vi "FormCalibra9-joao.vi"() -> ()   [LabVIEW 2014]
uses:
  testMachine.ctl
  mainMachine.ctl
  <vilib>/Instr/_visa.llb/VISA Configure Serial Port (Instr).vi
  <vilib>/express/express shared/transition.llb/Dynamic To Waveform Array.vi
  <vilib>/express/express signal manip/GetorSetDDTAttributes/Set DDT Attributes/SetT0.vi
  <vilib>/express/express shared/transition.llb/Waveform Array To Dynamic.vi
  <vilib>/express/express signal manip/GetorSetDDTAttributes/Set DDT Attributes/Set DDT Properties.xnode
panel:
  in  "VISA Serial Port":refnum<visa-resource-name>
  out "editDistance":dbl caption="Distancia (m)" format="%#_4f"
  in  "Lower level":dbl
  in  "hysteresis":dbl format="%.2p"
  in  "level":dbl format="%.2p"
  out "rpm":bool
  out "editTotalWaitLimit":u8
  out "editCountWaitLimit":u8
  out "ledWaitState":bool caption="Wait State"
  out "sliderWaitUpperTime":u8(slide) max=50 scale=0.0..100.0
  out "slideWaitLowerTime":u8(slide) max=30 scale=0.0..100.0
  out "slideWaitTime":u8(slide) scale=0.0..100.0
  out "labelTestTime":string caption="Tempo total de ensaio"
  in  "buttonAcquisition":bool
  in  "editSetWaitTime":u8 caption="Tempo entre ciclos (s)" step=1 format="%0d"
  in  "stop":bool
  out "ledAcquireState":bool caption="Acquire State"
  out "editTotalLowerLimit":u8
  out "editCountLowerLimit":u8
  out "editTotalUpperLimit":u8
  out "editCountUpperLimit":u8
  out "ledEnsaio 3":bool
  out "ledBrakeState":bool caption="Brake State"
  out "ledExitState":bool caption="Exit State"
  out "ledMotorState":bool caption="Motor State"
  out "ledInit2State":bool caption="Init State"
  out "ledBlockState":bool caption="Block State"
  out "ledRunningState":bool caption="Running State"
  out "ledReadyState":bool caption="Ready State"
  out "ledInitState":bool caption="Init State"
  out "mainMachine":T1
  out "testMachine":T2=enum."finish"
  in  "editSetPathToFile":path
  in  "buttonStop":bool
  in  "buttonStart":bool
  out "graphForce":dynamicdata(graph)
  in  "editOffsetForce":dbl caption="Tara" min=0.0 max=100.0 step=0.1
  in  "editSetForce":dbl caption="Fator de conversão"
  out "editForce":dbl caption="Força (Kgf)" format="%#_4f"
  out "graphSpeed":dynamicdata(graph)
  in  "editSetSpeed":dbl caption="Fator de conversão"
  out "editSpeed":dbl caption="Velocidade (km/h)" format="%#_4f"
  out "editEngineSpeed":dbl caption="Rotação (RPM)" format="%#_4f"
  in  "buttonMotor":bool
  in  "buttonBrake":bool
  in  "editSetWaitLowerTime":u8 caption="Tempo de espera (s)"
  in  "editSetWaitUpperTime":u8=3 caption="Tempo de espera (s)"
  in  "editSetNumberOfCycles":u16 caption="Número de ciclos" max=999 step=1 format="%0d"
  in  "editSetLowerLimit":u32 caption="Limite inferior (km/h)"
  in  "editSetUpperLimit":u32 caption="Limite superior (km/h)"
  out "editTempB":dbl caption="Temperatura B (ºC)"
  out "editTempA":dbl caption="Temperatura A (ºC)"
  in  "editSetTempRef":dbl caption="Offset referência" step=0.01 format="%#_2f"
  out "editTempRef":dbl caption="Referência (ºC)"
  out "ledMotor":bool
  out "ledBrake":bool
  out "ledEnsaio":bool
  out "labelTotalCycle":string
  out "labelCurrentCycle":string
  out "labelSystemTitle":string
  in  "editCurrCycleCtr":u32
  in  "velocidade 2":u32
  out "velocidade":u32
  # "Bancada de Frenagem - Ensaio"
  # "Ensaio"
  # "Temperatura"
  # "Rotação"
  # "Célula de Carga"
  # "Configurações do ensaio"
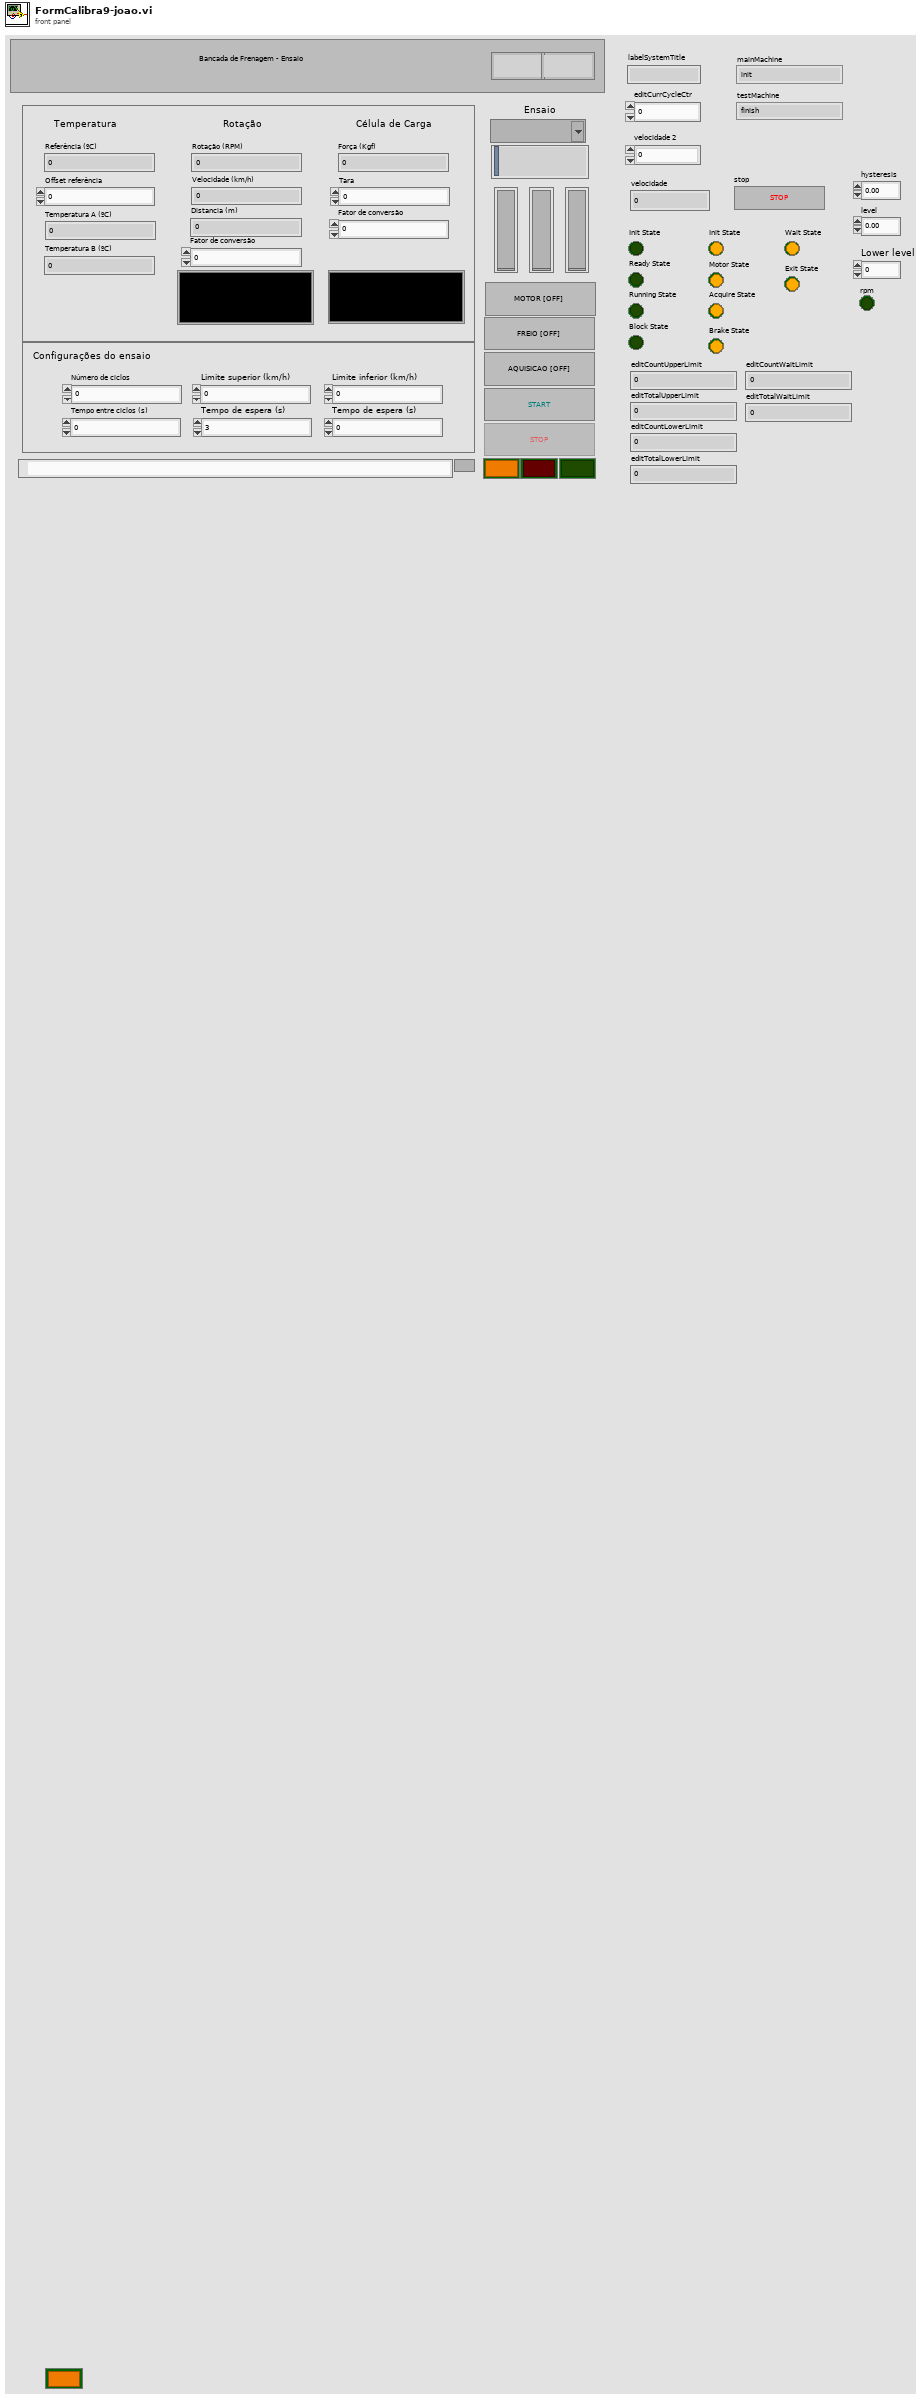
[diagram p1: front panel]
types:
  T1 = typedef "mainMachine.ctl" = enum16{"init", "ready", "running", "blocked", "finish"}
  T2 = typedef "testMachine.ctl" = enum16{"init", "motor", "motor acquire", "brake", "brake acquire", "wait ", "finish", "exit"}
  T3 = enum8{"Enabled", "Disabled", "Disabled and Grayed Out"}
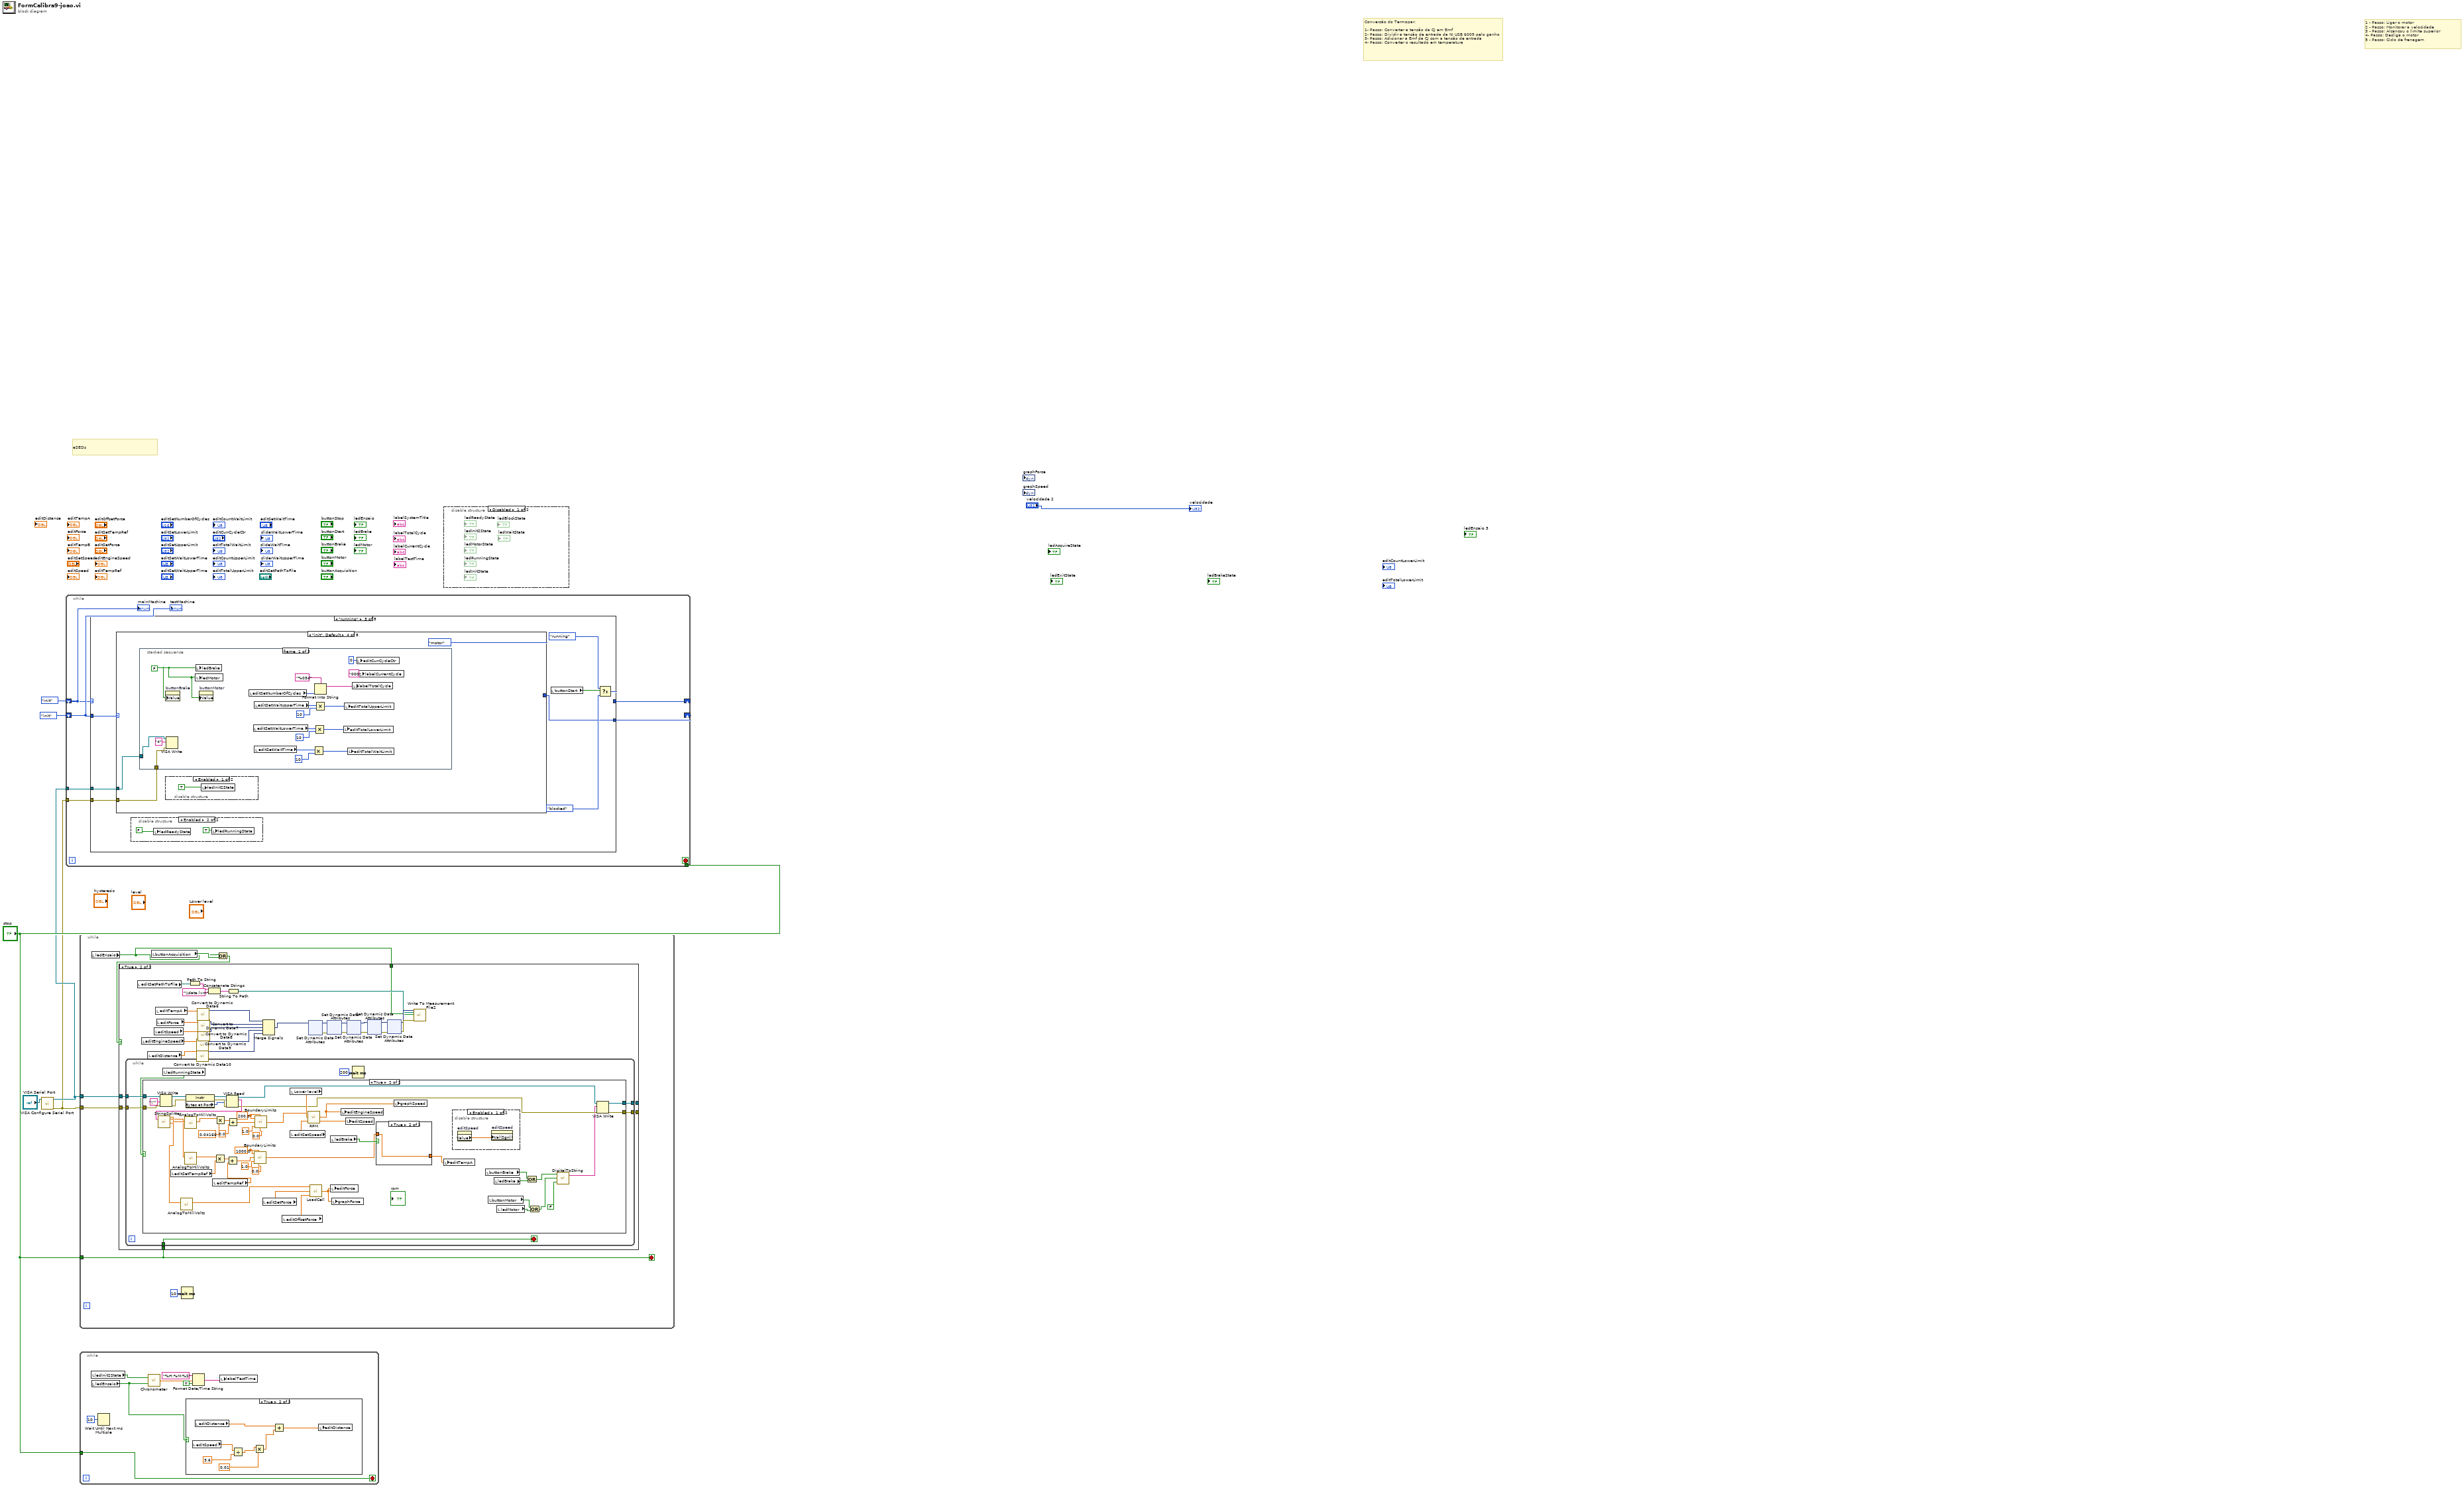
[diagram p0: block diagram]
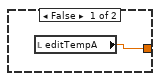
[diagram p6: hidden frame]
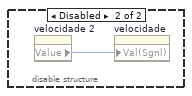
[diagram p7: hidden frame]
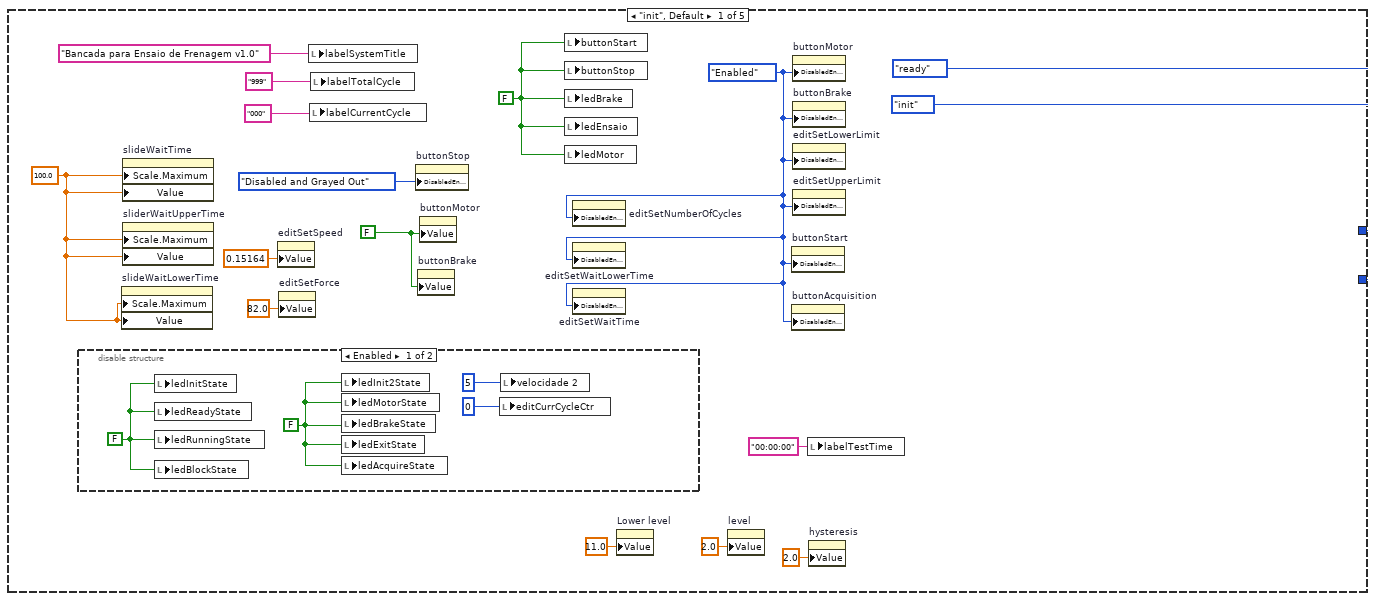
[diagram p8: hidden frame]
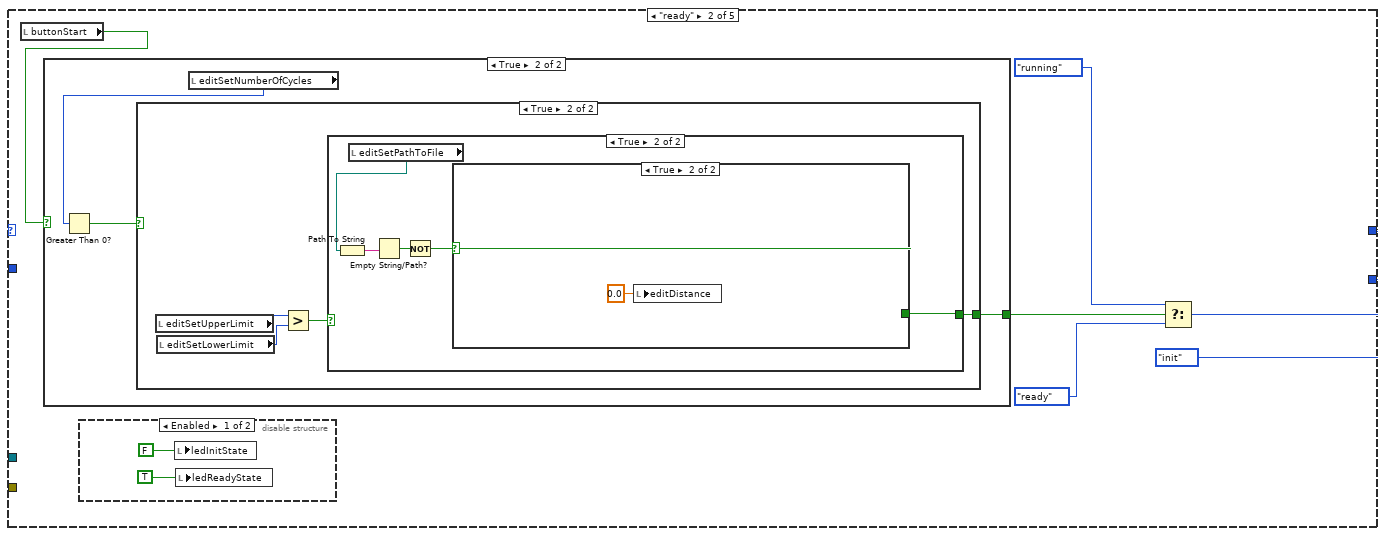
[diagram p10: hidden frame]
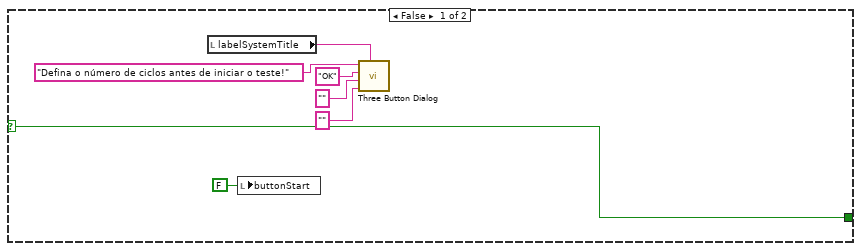
[diagram p13: hidden frame]
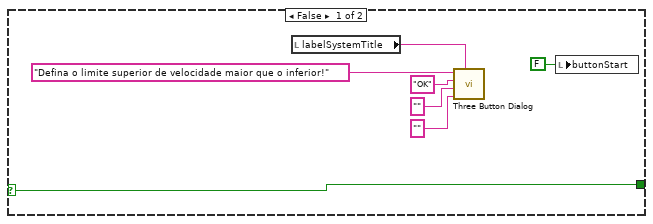
[diagram p14: hidden frame]
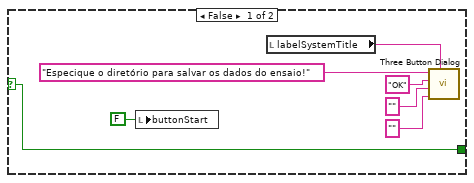
[diagram p15: hidden frame]
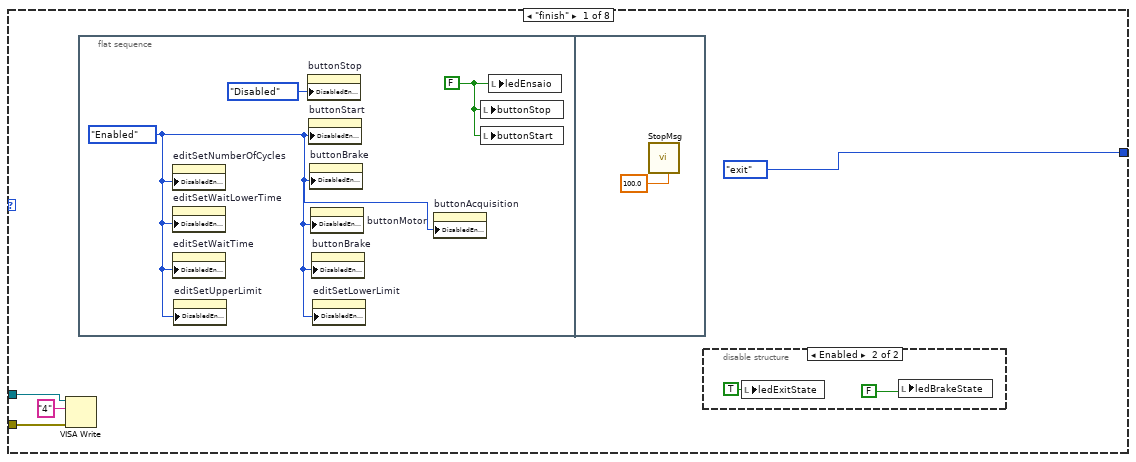
[diagram p17: hidden frame]
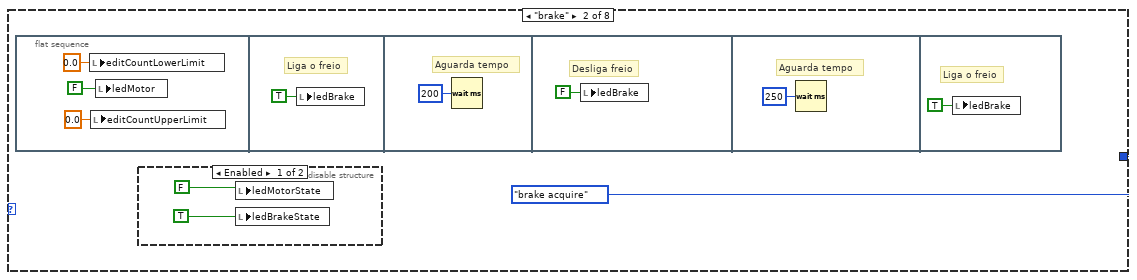
[diagram p19: hidden frame]
diagram:
  # "eSEDs"
  # "1 - Passo: Ligar o motor\n2 - Passo: Monitorar a velocidade\n3 - Passo: Alcancou o limite superior\n4- Passo: Desliga o motor\n5 - Passo: Ciclo de frenagem"
  # "Conversão do Termopar:\n\n1- Passo: Converter a tensão da CJ em Emf\n2- Passo: Dividir a tensão de entrada da NI USB 6009 pelo ganho\n3- Passo: Adicionar a Emf da CJ com a tensão de entrada\n4- Passo: Converter o resultado em temperatura"
  n1 = call-poly "VISA Configure Serial Port"("VISA resource name"="VISA Serial Port") -> ("VISA resource name out"=w3:refnum<visa-resource-name>, "error out"=w2:errorcluster)  [unwired: 13 in]
  n2 = while {
    shift-right: [w14] -> _
    shift-left: mainMachine."init" ("mainMachine") -> [w11]
    shift-right: [w13] -> _
    shift-left: testMachine."init" ("testMachine") -> [w12]
    tunnel: "stop" -> [w10]
    tunnel: w3 -> [w9]
    tunnel: w2 -> [w8]
    stop <- w10 stop-if-true
    n3 = case shown="\"running\"" w11 {
      tunnel: [mainMachine."ready" ("mainMachine") w35 w83 w235 mainMachine."finish" ("mainMachine")] -> w14
      tunnel: [testMachine."init" ("testMachine") testMachine."init" ("testMachine") w82 testMachine."init" ("testMachine") testMachine."init" ("testMachine")] -> w13
      tunnel: w12 -> [_ _ w81 _ _]
      tunnel: w9 -> [_ _ w80 _ _]
      tunnel: w8 -> [_ _ w79 _ _]
      frame "init", Default {
        w21 = 100.0 ("Scale.Range:Maximum")
        w22 = T3."Enabled" ("Disabled")
        w23 = FALSE ("buttonMotor")
        w29 = FALSE ("motor")
        n4 = disable-structure shown="Enabled" {
          frame Enabled {
            w31 = FALSE
            w32 = FALSE
            n5 = local write "ledInitState"(w32) -> ()
            n6 = local write "ledReadyState"(w32) -> ()
            n7 = local write "ledRunningState"(w32) -> ()
            n8 = local write "ledBlockState"(w32) -> ()
            n9 = local write "ledInit2State"(w31) -> ()
            n10 = local write "ledMotorState"(w31) -> ()
            n11 = local write "ledBrakeState"(w31) -> ()
            n12 = local write "ledExitState"(w31) -> ()
            n13 = local write "ledAcquireState"(w31) -> ()
            n14 = local write "editCurrCycleCtr"(u32 0 ("currentCycleCtr")) -> ()
            n15 = local write "velocidade 2"(u32 5 ("velocidade 2")) -> ()
          }
          frame Disabled {
          }
        }
        n16 = property on="slideWaitLowerTime" class="Slide (strict)"("Scale.Maximum"=w21, "Value"=w21) -> ()  [unwired: 2 in, 2 out]
        n17 = property on="slideWaitTime" class="Slide (strict)"("Scale.Maximum"=w21, "Value"=w21) -> ()  [unwired: 2 in, 2 out]
        n18 = property on="sliderWaitUpperTime" class="Slide (strict)"("Scale.Maximum"=w21, "Value"=w21) -> ()  [unwired: 2 in, 2 out]
        n19 = property on="editSetSpeed" class="DigNum (strict)"("Value"=0.15164 ("editSetSpeed")) -> ()  [unwired: 2 in, 2 out]
        n20 = property on="editSetForce" class="DigNum (strict)"("Value"=82.0 ("editSetForce")) -> ()  [unwired: 2 in, 2 out]
        n21 = local write "labelSystemTitle"("Bancada para Ensaio de Frenagem v1.0" ("systemTitle")) -> ()
        n22 = local write "labelCurrentCycle"("000" ("currentCycle")) -> ()
        n23 = local write "labelTotalCycle"("999" ("totalCycle")) -> ()
        n24 = property on="buttonStop" class="Bool (strict)"("DisabledEnum"=T3."Disabled and Grayed Out" ("Disabled")) -> ()  [unwired: 2 in, 2 out]
        n25 = property on="buttonBrake" class="Bool (strict)"("Value"=w23) -> ()  [unwired: 2 in, 2 out]
        n26 = property on="buttonMotor" class="Bool (strict)"("Value"=w23) -> ()  [unwired: 2 in, 2 out]
        n27 = local write "buttonStart"(w29) -> ()
        n28 = local write "buttonStop"(w29) -> ()
        n29 = local write "ledBrake"(w29) -> ()
        n30 = local write "ledEnsaio"(w29) -> ()
        n31 = local write "ledMotor"(w29) -> ()
        n32 = property on="editSetNumberOfCycles" class="DigNum (strict)"("DisabledEnum"=w22) -> ()  [unwired: 2 in, 2 out]
        n33 = property on="editSetWaitLowerTime" class="DigNum (strict)"("DisabledEnum"=w22) -> ()  [unwired: 2 in, 2 out]
        n34 = property on="editSetWaitTime" class="DigNum (strict)"("DisabledEnum"=w22) -> ()  [unwired: 2 in, 2 out]
        n35 = property on="Lower level" class="DigNum (strict)"("Value"=11.0 ("Lower level")) -> ()  [unwired: 2 in, 2 out]
        n36 = property on="level" class="DigNum (strict)"("Value"=2.0 ("level")) -> ()  [unwired: 2 in, 2 out]
        n37 = property on="buttonStart" class="Bool (strict)"("DisabledEnum"=w22) -> ()  [unwired: 2 in, 2 out]
        n38 = property on="buttonAcquisition" class="Bool (strict)"("DisabledEnum"=w22) -> ()  [unwired: 2 in, 2 out]
        n39 = property on="buttonMotor" class="Bool (strict)"("DisabledEnum"=w22) -> ()  [unwired: 2 in, 2 out]
        n40 = property on="buttonBrake" class="Bool (strict)"("DisabledEnum"=w22) -> ()  [unwired: 2 in, 2 out]
        n41 = property on="editSetLowerLimit" class="DigNum (strict)"("DisabledEnum"=w22) -> ()  [unwired: 2 in, 2 out]
        n42 = property on="editSetUpperLimit" class="DigNum (strict)"("DisabledEnum"=w22) -> ()  [unwired: 2 in, 2 out]
        n43 = local write "labelTestTime"("00:00:00" ("labelTestTime")) -> ()
        n44 = property on="hysteresis" class="DigNum (strict)"("Value"=2.0 ("hysteresis")) -> ()  [unwired: 2 in, 2 out]
      }
      frame "ready" {
        n45 = local read "buttonStart"() -> (w38:bool)
        n46 = case shown="True" w38 {
          selector: w38 -> [w43 _]
          tunnel: [w43 w44] -> w37
          frame False {
          }
          frame True {
            n47 = local read "editSetNumberOfCycles"() -> (w45:u16)
            n48 = Greater Than 0?(x=w45) -> (x > 0?=w46:bool)
            n49 = case shown="True" w46 {
              selector: w46 -> [w53 _]
              tunnel: [w53 w54] -> w44
              frame False {
                n50 = local read "labelSystemTitle"() -> (w48:string)
                n51 = local write "buttonStart"(FALSE ("startButton")) -> ()
                n52 = call <vilib>:"Three Button Dialog.vi"("Window Title (\"\")"=w48, "Right Button Text (\"Cancel\")"="" ("Right Button Text (\"Cancel\")"), "Center Button Text (\"No\")"="" ("Center Button Text (\"No\")"), "Left Button Text (\"Yes\")"="OK" ("Left Button Text (\"Yes\")"), "message"="Defina o número de ciclos antes de iniciar o teste!") -> ()  [unwired: 6 in, 1 out]
              }
              frame True {
                n53 = local read "editSetUpperLimit"() -> (w56:u32)
                n54 = local read "editSetLowerLimit"() -> (w55:u32)
                n55 = Greater?(x=w56, y=w55) -> (0:w57:bool)
                n56 = case shown="True" w57 {
                  selector: w57 -> [w64 _]
                  tunnel: [w64 w67] -> w54
                  frame False {
                    n57 = local read "labelSystemTitle"() -> (w59:string)
                    n58 = call <vilib>:"Three Button Dialog.vi"("Window Title (\"\")"=w59, "Right Button Text (\"Cancel\")"="" ("Right Button Text (\"Cancel\")"), "Center Button Text (\"No\")"="" ("Center Button Text (\"No\")"), "Left Button Text (\"Yes\")"="OK" ("Left Button Text (\"Yes\")"), "message"="Defina o limite superior de velocidade maior que o inferior!") -> ()  [unwired: 6 in, 1 out]
                    n59 = local write "buttonStart"(FALSE ("startButton")) -> ()
                  }
                  frame True {
                    n60 = local read "editSetPathToFile"() -> (w69:path)
                    n61 = Path To String(path=w69) -> (string=w68:string)
                    n62 = Empty String/Path?(string/path=w68) -> (empty?=w66:bool)
                    n63 = Not(x=w66) -> (.not. x?=w65:bool)
                    n64 = case shown="True" w65 {
                      selector: w65 -> [w76 w78]
                      tunnel: [w76 w78] -> w67
                      frame False {
                        n65 = local write "buttonStart"(FALSE ("startButton")) -> ()
                        n66 = local read "labelSystemTitle"() -> (w71:string)
                        n67 = call <vilib>:"Three Button Dialog.vi"("Window Title (\"\")"=w71, "Right Button Text (\"Cancel\")"="" ("Right Button Text (\"Cancel\")"), "Center Button Text (\"No\")"="" ("Center Button Text (\"No\")"), "Left Button Text (\"Yes\")"="OK" ("Left Button Text (\"Yes\")"), "message"="Especique o diretório para salvar os dados do ensaio!") -> ()  [unwired: 6 in, 1 out]
                      }
                      frame True {
                        n68 = local write "editDistance"(0.0 ("editDistance")) -> ()
                      }
                    }
                  }
                }
              }
            }
          }
        }
        n69 = disable-structure shown="Enabled" {
          frame Enabled {
            n70 = local write "ledInitState"(FALSE ("ledReady")) -> ()
            n71 = local write "ledReadyState"(TRUE ("ledReady")) -> ()
          }
          frame Disabled {
          }
        }
        n72 = Select(t=mainMachine."running" ("mainMachine"), s=w37, f=mainMachine."ready" ("mainMachine")) -> (s? t:f=w35:T1)
      }
      frame "running" {
        n73 = case shown="\"init\", Default" w81 {
          tunnel: [testMachine."exit" ("testMachine") testMachine."brake acquire" ("testMachine") testMachine."motor acquire" ("testMachine") testMachine."motor" ("testMachine") w165 w185 testMachine."exit" ("testMachine") w218] -> w82
          tunnel: w80 -> [w90 _ _ w129 _ _ _ _]
          tunnel: w79 -> [w89 _ _ w128 _ _ _ _]
          frame "finish" {
            n74 = VISA Write(VISA resource name=w90, write buffer="4", error in (no error)=w89) -> ()  [unwired: 3 out]
            n75 = flat-sequence {
              frame #0 {
                w96 = FALSE ("ledReady")
                w95 = T3."Enabled" ("Disabled")
                n76 = property on="editSetNumberOfCycles" class="DigNum (strict)"("DisabledEnum"=w95) -> ()  [unwired: 2 in, 2 out]
                n77 = property on="editSetWaitLowerTime" class="DigNum (strict)"("DisabledEnum"=w95) -> ()  [unwired: 2 in, 2 out]
                n78 = property on="editSetWaitTime" class="DigNum (strict)"("DisabledEnum"=w95) -> ()  [unwired: 2 in, 2 out]
                n79 = property on="editSetUpperLimit" class="DigNum (strict)"("DisabledEnum"=w95) -> ()  [unwired: 2 in, 2 out]
                n80 = property on="buttonStop" class="Bool (strict)"("DisabledEnum"=T3."Disabled" ("Disabled")) -> ()  [unwired: 2 in, 2 out]
                n81 = property on="buttonStart" class="Bool (strict)"("DisabledEnum"=w95) -> ()  [unwired: 2 in, 2 out]
                n82 = property on="buttonBrake" class="Bool (strict)"("DisabledEnum"=w95) -> ()  [unwired: 2 in, 2 out]
                n83 = property on="buttonMotor" class="Bool (strict)"("DisabledEnum"=w95) -> ()  [unwired: 2 in, 2 out]
                n84 = property on="buttonBrake" class="Bool (strict)"("DisabledEnum"=w95) -> ()  [unwired: 2 in, 2 out]
                n85 = property on="editSetLowerLimit" class="DigNum (strict)"("DisabledEnum"=w95) -> ()  [unwired: 2 in, 2 out]
                n86 = property on="buttonAcquisition" class="Bool (strict)"("DisabledEnum"=w95) -> ()  [unwired: 2 in, 2 out]
                n87 = local write "buttonStop"(w96) -> ()
                n88 = local write "buttonStart"(w96) -> ()
                n89 = local write "ledEnsaio"(w96) -> ()
              }
              frame #1 {
                n90 = call "StopMsg.vi"("Max Value (100)"=100.0) -> ()  [unwired: 8 in, 2 out]
              }
            }
            n91 = disable-structure shown="Enabled" {
              frame Disabled {
              }
              frame Enabled {
                n92 = local write "ledExitState"(TRUE ("ledReady")) -> ()
                n93 = local write "ledBrakeState"(FALSE ("ledReady")) -> ()
              }
            }
          }
          frame "brake" {
            n94 = flat-sequence {
              frame #0 {
                n95 = local write "editCountLowerLimit"(0.0 ("editCountUpperLimit")) -> ()
                n96 = local write "editCountUpperLimit"(0.0 ("editCountUpperLimit")) -> ()
                n97 = local write "ledMotor"(FALSE ("motor")) -> ()
              }
              frame #1 {
                # "Liga o freio"
                n98 = local write "ledBrake"(TRUE ("freio")) -> ()
              }
              frame #2 {
                # "Aguarda tempo"
                n99 = Wait (ms)(milliseconds to wait=u32 200) -> ()  [unwired: 1 out]
              }
              frame #3 {
                # "Desliga freio"
                n100 = local write "ledBrake"(FALSE ("freio")) -> ()
              }
              frame #4 {
                # "Aguarda tempo"
                n101 = Wait (ms)(milliseconds to wait=u32 250) -> ()  [unwired: 1 out]
              }
              frame #5 {
                # "Liga o freio"
                n102 = local write "ledBrake"(TRUE ("freio")) -> ()
              }
            }
            n103 = disable-structure shown="Enabled" {
              frame Enabled {
                n104 = local write "ledMotorState"(FALSE ("ledReady")) -> ()
                n105 = local write "ledBrakeState"(TRUE ("ledReady")) -> ()
              }
              frame Disabled {
              }
            }
          }
          frame "motor" {
            n106 = flat-sequence {
              frame #0 {
                n107 = local read "editCurrCycleCtr"() -> (w115:u32)
                n108 = Increment(x=w115) -> (x+1=w114:u32)
                n109 = local write "editCurrCycleCtr"(w114) -> ()
              }
              frame #1 {
                n110 = local read "editCurrCycleCtr"() -> (w122:u32)
                n111 = local read "editTotalWaitLimit"() -> (w116:u8)
                n112 = local read "editTotalUpperLimit"() -> (w118:u8)
                n113 = local read "editTotalLowerLimit"() -> (w117:u8)
                n114 = local write "editCountLowerLimit"(u8 0 ("editCountLowerLimit")) -> ()
                n115 = local write "editCountWaitLimit"(u8 0 ("editCountWaitLimit")) -> ()
                n116 = local write "editCountUpperLimit"(u8 0 ("editCountUpperLimit")) -> ()
                n117 = Format Into String(format string="%03d", w122) -> (resulting string=w123:string)  [unwired: 2 in, 1 out]
                n118 = property on="sliderWaitUpperTime" class="Slide (strict)"("Value"=w118) -> ()  [unwired: 2 in, 2 out]
                n119 = property on="slideWaitLowerTime" class="Slide (strict)"("Value"=w117) -> ()  [unwired: 2 in, 2 out]
                n120 = property on="slideWaitTime" class="Slide (strict)"("Value"=w116) -> ()  [unwired: 2 in, 2 out]
                n121 = local write "labelCurrentCycle"(w123) -> ()
              }
              frame #2 {
                # "- Liga o motor"
                n122 = local write "ledMotor"(TRUE ("motor")) -> ()
                n123 = property on="buttonStop" class="Bool (strict)"("DisabledEnum"=T3."Enabled" ("Disabled")) -> ()  [unwired: 2 in, 2 out]
                n124 = property on="buttonStart" class="Bool (strict)"("DisabledEnum"=T3."Disabled and Grayed Out" ("Disabled")) -> ()  [unwired: 2 in, 2 out]
              }
            }
            n125 = disable-structure shown="Enabled" {
              frame Enabled {
                n126 = local write "ledInit2State"(FALSE ("ledReady")) -> ()
                n127 = local write "ledBrakeState"(FALSE ("ledReady")) -> ()
                n128 = local write "ledMotorState"(TRUE ("ledReady")) -> ()
              }
              frame Disabled {
              }
            }
          }
          frame "init", Default {
            n129 = stacked-sequence {
              tunnel: w129 -> [w133 _ _]
              tunnel: w128 -> [w132 _ _]
              frame #0 {
                w140 = FALSE ("ensaio")
                n130 = property on="buttonBrake" class="Bool (strict)"("Value"=w140) -> ()  [unwired: 2 in, 2 out]
                n131 = VISA Write(VISA resource name=w133, write buffer="4", error in (no error)=w132) -> ()  [unwired: 3 out]
                n132 = local write "ledMotor"(w140) -> ()
                n133 = local write "ledBrake"(w140) -> ()
                n134 = property on="buttonMotor" class="Bool (strict)"("Value"=w140) -> ()  [unwired: 2 in, 2 out]
                n135 = local read "editSetNumberOfCycles"() -> (w147:u16)
                n136 = local read "editSetWaitLowerTime"() -> (w141:u8)
                n137 = local read "editSetWaitUpperTime"() -> (w144:u8)
                n138 = local read "editSetWaitTime"() -> (w135:u8)
                n139 = Multiply(x=w135, y=u32 10) -> (x*y=w136:u32)
                n140 = Multiply(x=w141, y=u32 10) -> (x*y=w139:u32)
                n141 = Format Into String(format string="%03d", w147) -> (resulting string=w148:string)  [unwired: 2 in, 1 out]
                n142 = Multiply(x=w144, y=u32 10) -> (x*y=w138:u32)
                n143 = local write "editTotalLowerLimit"(w139) -> ()
                n144 = local write "editTotalUpperLimit"(w138) -> ()
                n145 = local write "editTotalWaitLimit"(w136) -> ()
                n146 = local write "labelTotalCycle"(w148) -> ()
                n147 = local write "editCurrCycleCtr"(u32 0 ("currentCycleCtr")) -> ()
                n148 = local write "labelCurrentCycle"("000" ("currentCycle")) -> ()
              }
              frame #1 {
                w156 = T3."Disabled" ("Disabled")
                n149 = property on="editSetNumberOfCycles" class="DigNum (strict)"("DisabledEnum"=w156) -> ()  [unwired: 2 in, 2 out]
                n150 = property on="editSetWaitLowerTime" class="DigNum (strict)"("DisabledEnum"=w156) -> ()  [unwired: 2 in, 2 out]
                n151 = property on="editSetWaitTime" class="DigNum (strict)"("DisabledEnum"=w156) -> ()  [unwired: 2 in, 2 out]
                n152 = local read "editTotalUpperLimit"() -> (w159:u8)
                n153 = property on="sliderWaitUpperTime" class="Slide (strict)"("Scale.Maximum"=w159, "Scale.Minimum"=0.0 ("Scale.Range:Minimum"), "Scale.Increment"=1.0 ("Scale.Range:Increment"), "Value"=w159) -> ()  [unwired: 2 in, 2 out]
                n154 = property on="buttonAcquisition" class="Bool (strict)"("DisabledEnum"=w156) -> ()  [unwired: 2 in, 2 out]
                n155 = local read "editTotalLowerLimit"() -> (w153:u8)
                n156 = property on="slideWaitLowerTime" class="Slide (strict)"("Scale.Maximum"=w153, "Scale.Minimum"=0.0 ("Scale.Range:Minimum"), "Scale.Increment"=1.0 ("Scale.Range:Increment"), "Value"=w153) -> ()  [unwired: 2 in, 2 out]
                n157 = local read "editTotalWaitLimit"() -> (w150:u8)
                n158 = property on="slideWaitTime" class="Slide (strict)"("Scale.Maximum"=w150, "Scale.Minimum"=0.0 ("Scale.Range:Minimum"), "Scale.Increment"=1.0 ("Scale.Range:Increment"), "Value"=w150) -> ()  [unwired: 2 in, 2 out]
                n159 = call "StarMsg.vi"("Show"=TRUE, "Max Value (100)"=100.0) -> ()  [unwired: 7 in, 2 out]
                n160 = property on="buttonMotor" class="Bool (strict)"("DisabledEnum"=w156) -> ()  [unwired: 2 in, 2 out]
                n161 = property on="buttonBrake" class="Bool (strict)"("DisabledEnum"=w156) -> ()  [unwired: 2 in, 2 out]
                n162 = property on="editSetLowerLimit" class="DigNum (strict)"("DisabledEnum"=w156) -> ()  [unwired: 2 in, 2 out]
                n163 = property on="editSetUpperLimit" class="DigNum (strict)"("DisabledEnum"=w156) -> ()  [unwired: 2 in, 2 out]
              }
              frame #2 {
                n164 = local write "ledEnsaio"(TRUE ("ensaio")) -> ()
              }
            }
            n165 = disable-structure shown="Enabled" {
              frame Enabled {
                n166 = local write "ledInit2State"(TRUE ("ledReady")) -> ()
              }
              frame Disabled {
              }
            }
          }
          frame "motor acquire" {
            n167 = disable-structure shown="Enabled" {
              frame Enabled {
                n168 = local read "ledAcquireState"() -> (w174:bool)
                n169 = Not(x=w174) -> (.not. x?=w173:bool)
                n170 = local write "ledAcquireState"(w173) -> ()
              }
              frame Disabled {
              }
            }
            n171 = Wait (ms)(milliseconds to wait=u32 100) -> ()  [unwired: 1 out]
            n172 = disable-structure shown="Enabled" {
              disable-tunnel: [w171 w172] -> w164
              frame Enabled {
                n173 = property on="editSpeed" class="DigNum (strict)"() -> ("Value"=w171:dbl)  [unwired: 2 in, 2 out]
              }
              frame Disabled {
                n174 = property on="velocidade" class="DigNum (strict)"() -> ("Value"=w172:u32)  [unwired: 2 in, 2 out]
              }
            }
            n175 = property on="editSetUpperLimit" class="DigNum (strict)"() -> ("Value"=w163:u32)  [unwired: 2 in, 2 out]
            n176 = Greater Or Equal?(x=w164, y=w163) -> (x >= y?=w169:bool)
            n177 = case shown="True" w169 {
              selector: w169 -> [w175 _]
              tunnel: [w175 w176] -> w168
              frame False {
              }
              frame True {
                n178 = flat-sequence {
                  tunnel: [w181] -> w176
                  frame #0 {
                    n179 = local read "editCountUpperLimit"() -> (w179:u8)
                    n180 = Increment(x=w179) -> (x+1=w177:u8)
                    n181 = local write "editCountUpperLimit"(w177) -> ()
                    n182 = local read "editTotalUpperLimit"() -> (w178:u8)
                    n183 = Subtract(x=w178, y=w177) -> (x-y=w180:u8)
                    n184 = property on="sliderWaitUpperTime" class="Slide (strict)"("Value"=w180) -> ()  [unwired: 2 in, 2 out]
                  }
                  frame #1 {
                    n185 = local read "editCountUpperLimit"() -> (w183:u8)
                    n186 = local read "editTotalUpperLimit"() -> (w182:u8)
                    n187 = Greater Or Equal?(x=w183, y=w182) -> (x >= y?=w181:bool)
                  }
                }
              }
            }
            n188 = Select(t=testMachine."brake" ("testMachine"), s=w168, f=testMachine."motor acquire" ("testMachine")) -> (s? t:f=w165:T2)
          }
          frame "brake acquire" {
            n189 = disable-structure shown="Enabled" {
              frame Enabled {
                n190 = local read "ledAcquireState"() -> (w193:bool)
                n191 = Not(x=w193) -> (.not. x?=w192:bool)
                n192 = local write "ledAcquireState"(w192) -> ()
              }
              frame Disabled {
              }
            }
            n193 = Wait (ms)(milliseconds to wait=u32 100) -> ()  [unwired: 1 out]
            n194 = disable-structure shown="Enabled" {
              disable-tunnel: [w194 w195] -> w184
              frame Enabled {
                n195 = property on="editSpeed" class="DigNum (strict)"() -> ("Value"=w194:dbl)  [unwired: 2 in, 2 out]
              }
              frame Disabled {
                n196 = property on="velocidade" class="DigNum (strict)"() -> ("Value"=w195:u32)  [unwired: 2 in, 2 out]
              }
            }
            n197 = property on="editSetLowerLimit" class="DigNum (strict)"() -> ("Value"=w186:u32)  [unwired: 2 in, 2 out]
            n198 = Less Or Equal?(x=w184, y=w186) -> (x <= y?=w190:bool)
            n199 = case shown="True" w190 {
              selector: w190 -> [w196 _]
              tunnel: [w196 w197] -> w188
              frame False {
              }
              frame True {
                n200 = flat-sequence {
                  tunnel: [w203] -> w198
                  tunnel: w198 -> [w207]
                  tunnel: [w206] -> w197
                  frame #0 {
                    n201 = local read "editCountLowerLimit"() -> (w202:u8)
                    n202 = Increment(x=w202) -> (x+1=w201:u8)
                    n203 = local write "editCountLowerLimit"(w201) -> ()
                    n204 = local read "editTotalLowerLimit"() -> (w200:u8)
                    n205 = Subtract(x=w200, y=w201) -> (x-y=w199:u8)
                    n206 = property on="slideWaitLowerTime" class="Slide (strict)"("Value"=w199) -> ()  [unwired: 2 in, 2 out]
                  }
                  frame #1 {
                    n207 = local read "editCountLowerLimit"() -> (w205:u8)
                    n208 = local read "editTotalLowerLimit"() -> (w204:u8)
                    n209 = Greater Or Equal?(x=w205, y=w204) -> (x >= y?=w203:bool)
                  }
                  frame #2 {
                    n210 = case shown="True" w207 {
                      selector: w207 -> [w208 w209]
                      tunnel: [w208 w209] -> w206
                      frame False {
                      }
                      frame True {
                        # "- Desliga o freio"
                        n211 = local write "ledBrake"(FALSE ("freio")) -> ()
                      }
                    }
                  }
                }
              }
            }
            n212 = Select(t=testMachine."wait " ("testMachine"), s=w188, f=testMachine."brake acquire" ("testMachine")) -> (s? t:f=w185:T2)
          }
          frame "exit" {
          }
          frame "wait " {
            # "- Aguarda 0.5s \n- Atualiza o numero de ciclos"
            n213 = flat-sequence {
              tunnel: [w224] -> w212
              frame #0 {
                n214 = local read "editCountWaitLimit"() -> (w220:u8)
                n215 = Increment(x=w220) -> (x+1=w221:u8)
                n216 = local write "editCountWaitLimit"(w221) -> ()
                n217 = local read "editTotalWaitLimit"() -> (w223:u8)
                n218 = Subtract(x=w223, y=w221) -> (x-y=w222:u8)
                n219 = property on="slideWaitTime" class="Slide (strict)"("Value"=w222) -> ()  [unwired: 2 in, 2 out]
              }
              frame #1 {
                n220 = local read "editCountWaitLimit"() -> (w226:u8)
                n221 = local read "editTotalWaitLimit"() -> (w225:u8)
                n222 = Greater Or Equal?(x=w226, y=w225) -> (x >= y?=w224:bool)
              }
            }
            n223 = disable-structure shown="Enabled" {
              frame Enabled {
                n224 = local read "ledWaitState"() -> (w233:bool)
                n225 = Not(x=w233) -> (.not. x?=w232:bool)
                n226 = local write "ledBrakeState"(FALSE ("ledBrakeState")) -> ()
                n227 = local write "ledWaitState"(w232) -> ()
              }
              frame Disabled {
              }
            }
            n228 = Wait (ms)(milliseconds to wait=u32 100) -> ()  [unwired: 1 out]
            n229 = case shown="True" w212 {
              selector: w212 -> [w227 _]
              tunnel: [w227 w231] -> w213
              frame False {
              }
              frame True {
                n230 = local read "editSetNumberOfCycles"() -> (w229:u16)
                n231 = local read "editCurrCycleCtr"() -> (w228:u32)
                n232 = Greater Or Equal?(x=w228, y=w229) -> (x >= y?=w231:bool)
                n233 = Not(x=w231) -> (.not. x?=w230:bool)
                n234 = local write "ledEnsaio"(w230) -> ()
              }
            }
            n235 = Select(t=testMachine."motor" ("testMachine"), s=w212, f=testMachine."wait " ("testMachine")) -> (s? t:f=w214:T2)
            n236 = Select(t=testMachine."finish" ("testMachine"), s=w213, f=w214) -> (s? t:f=w218:T2)
          }
        }
        n237 = disable-structure shown="Enabled" {
          frame Disabled {
          }
          frame Enabled {
            n238 = local write "ledReadyState"(FALSE ("ledReady")) -> ()
            n239 = local write "ledRunningState"(TRUE ("ledReady")) -> ()
          }
        }
        n240 = local read "buttonStart"() -> (w86:bool)
        n241 = Select(t=mainMachine."running" ("mainMachine"), s=w86, f=mainMachine."blocked" ("mainMachine")) -> (s? t:f=w83:T1)
      }
      frame "blocked" {
        n242 = local read "buttonStart"() -> (w239:bool)
        n243 = Select(t=mainMachine."ready" ("mainMachine"), s=w239, f=mainMachine."blocked" ("mainMachine")) -> (s? t:f=w235:T1)
        n244 = local write "ledRunningState"(FALSE ("ledReady")) -> ()
        n245 = local write "ledBlockState"(TRUE ("ledReady")) -> ()
      }
      frame "finish" {
        n246 = local write "ledBlockState"(FALSE ("ledReady")) -> ()
      }
    }
    "mainMachine" <- w11
    "testMachine" <- w12
  }
  n247 = while {
    tunnel: "stop" -> [w252]
    stop <- w252 stop-if-true
    n248 = local read "ledInit2State"() -> (w247:bool)
    n249 = local read "ledEnsaio"() -> (w245:bool)
    n250 = Wait Until Next ms Multiple(millisecond multiple=u32 10) -> ()  [unwired: 1 out]
    n251 = call "Chronometer.vi"("start"=w245, "reset"=w247) -> ("Time"=w251:dbl)
    n252 = case shown="True" w245 {
      frame False {
      }
      frame True {
        n253 = local read "editSpeed"() -> (w257:dbl)
        n254 = local read "editDistance"() -> (w259:dbl)
        n255 = Divide(x=w257, y=3.6) -> (x/y=w255:dbl)
        n256 = Multiply(x=w255, y=0.01) -> (x*y=w254:dbl)
        n257 = Add(x=w259, y=w254) -> (x+y=w253:dbl)
        n258 = local write "editDistance"(w253) -> ()
      }
    }
    n259 = Format Date/Time String(time format string (%c)="%H:%M:%S", seconds (now)=w251, UTC format=TRUE) -> (date/time string=w248:string)
    n260 = local write "labelTestTime"(w248) -> ()
  }
  n261 = while {
    tunnel: "stop" -> [w266]
    tunnel: w3 -> [w261]
    tunnel: w2 -> [w260]
    stop <- w266 stop-if-true
    n262 = local read "ledEnsaio"() -> (w263:bool)
    n263 = local read "buttonAcquisition"() -> (w265:bool)
    n264 = Wait (ms)(milliseconds to wait=u32 10) -> ()  [unwired: 1 out]
    n265 = Or(x=w263, y=w265) -> (x .or. y?=w264:bool)
    n266 = case shown="True" w264 {
      tunnel: w266 -> [_ w269]
      tunnel: w263 -> [_ w278]
      tunnel: w261 -> [w268 w273]
      tunnel: w260 -> [w267 w272]
      tunnel: [w268 w271] -> _
      tunnel: [w267 w270] -> _
      frame False {
      }
      frame True {
        n267 = while {
          tunnel: w273 -> [w307]
          tunnel: w272 -> [w306]
          tunnel: [w305] -> w271
          tunnel: [w304] -> w270
          tunnel: w269 -> [w303]
          stop <- w303 stop-if-true
          n268 = local read "ledRunningState"() -> (w301:bool)
          n269 = case shown="True" w301 {
            tunnel: w307 -> [w309 w323]
            tunnel: w306 -> [w308 w322]
            tunnel: [w309 w319] -> w305
            tunnel: [w308 w318] -> w304
            frame False {
            }
            frame True {
              w347 = 1000.0
              w351 = 200.0
              n270 = VISA Write(VISA resource name=w323, write buffer="\"", error in (no error)=w322) -> (VISA resource name out=w329:refnum<visa-resource-name>, error out=w328:errorcluster)  [unwired: 1 out]
              n271 = local read "editSetTempRef"() -> (w339:dbl)
              n272 = property class="Instr"(reference=w329, error in=w328) -> (reference out=w332:refnum<visa-resource-name>, error out=w331:errorcluster, "Bytes at Port"=w330:u32)
              n273 = local read "editTempRef"() -> (w338:dbl)
              n274 = VISA Read(VISA resource name=w332, byte count=w330, error in (no error)=w331) -> (VISA resource name out=w321:refnum<visa-resource-name>, read buffer=w324:string, error out=w320:errorcluster)  [unwired: 1 out]
              n275 = call "StringSplitter.vi"("Input String"=w324) -> ("S0"=w356:dbl, "S1"=w341:dbl, "S3"=w326:dbl)  [unwired: 11 in, 5 out]
              n276 = call "AnalogToMiliVolts.vi"("Input"=w326) -> ("Output"=w325:dbl)  [unwired: 10 in]
              n277 = call "AnalogToMiliVolts.vi"("Input"=w356) -> ("Output"=w355:dbl)  [unwired: 10 in]
              n278 = call "AnalogToMiliVolts.vi"("Input"=w341) -> ("Output"=w342:dbl)  [unwired: 10 in]
              n279 = Multiply(x=w342, y=w339) -> (x*y=w343:dbl)
              n280 = Multiply(x=w355, y=0.04166) -> (x*y=w352:dbl)
              n281 = Add(x=w343, y=w338) -> (x+y=w344:dbl)
              n282 = Add(x=w352, y=0.0) -> (x+y=w350:dbl)
              n283 = call "BoundaryLimits.vi"("UpperLimit"=w347, "UpperValue"=w347, "Input"=w344, "LowerLimit"=1.0, "LowerValue"=0.0) -> ("Output"=w335:dbl)
              n284 = call "BoundaryLimits.vi"("UpperLimit"=w351, "UpperValue"=w351, "Input"=w350, "LowerLimit"=1.0, "LowerValue"=0.0) -> ("Output"=w340:dbl)
              n285 = local read "editSetForce"() -> (w360:dbl)
              n286 = local read "editOffsetForce"() -> (w361:dbl)
              n287 = local read "Lower level"() -> (w357:dbl)
              n288 = local read "editSetSpeed"() -> (w358:dbl)
              n289 = call "RPM.vi"("factor"=w358, "Lower level"=w357, "data"=w340) -> ("km/h"=w359:dbl, "RPM"=w334:dbl)  [unwired: 1 out]
              n290 = call "LoadCell.vi"("tara"=w361, "factor"=w360, "data"=w325) -> ("force (Kgf)"=w333:dbl)
              n291 = local read "ledBrake"() -> (w337:bool)
              n292 = local write "editForce"(w333) -> ()
              n293 = local write "graphForce"(w333) -> ()
              n294 = local write "editEngineSpeed"(w334) -> ()
              n295 = local write "editSpeed"(w359) -> ()
              n296 = case shown="True" w337 {
                tunnel: w335 -> [_ w363]
                tunnel: [w362 w363] -> w336
                frame False {
                  n297 = local read "editTempA"() -> (w362:dbl)
                }
                frame True {
                }
              }
              n298 = local write "graphSpeed"(w334) -> ()
              n299 = local write "editTempA"(w336) -> ()
              n300 = disable-structure shown="Enabled" {
                frame Enabled {
                  n301 = property on="editSpeed" class="DigNum (strict)"() -> ("Value"=w364:dbl)  [unwired: 2 in, 2 out]
                  n302 = property on="editSpeed" class="DigNum (strict)"("Val(Sgnl)"=w364) -> ()  [unwired: 2 in, 2 out]
                }
                frame Disabled {
                  n303 = property on="velocidade 2" class="DigNum (strict)"() -> ("Value"=w365:u32)  [unwired: 2 in, 2 out]
                  n304 = property on="velocidade" class="DigNum (strict)"("Val(Sgnl)"=w365) -> ()  [unwired: 2 in, 2 out]
                }
              }
              n305 = local read "buttonBrake"() -> (w315:bool)
              n306 = local read "buttonMotor"() -> (w317:bool)
              n307 = local read "ledBrake"() -> (w314:bool)
              n308 = local read "ledMotor"() -> (w316:bool)
              n309 = Or(x=w315, y=w314) -> (x .or. y?=w312:bool)
              n310 = Or(x=w317, y=w316) -> (x .or. y?=w311:bool)
              n311 = call "DigitalToString.vi"("D3"=FALSE, "D2"=w311, "D1"=w312) -> ("String"=w313:string)  [unwired: 1 out]
              n312 = VISA Write(VISA resource name=w321, write buffer=w313, error in (no error)=w320) -> (VISA resource name out=w319:refnum<visa-resource-name>, error out=w318:errorcluster)  [unwired: 1 out]
            }
          }
          n313 = Wait (ms)(milliseconds to wait=u32 200) -> ()  [unwired: 1 out]
        }
        n314 = local read "editSetPathToFile"() -> (w280:path)
        n315 = local read "editEngineSpeed"() -> (w276:dbl)
        n316 = local read "editDistance"() -> (w277:dbl)
        n317 = local read "editSpeed"() -> (w274:dbl)
        n318 = local read "editTempA"() -> (w292:dbl)
        n319 = local read "editForce"() -> (w275:dbl)
        n320 = Path To String(path=w280) -> (string=w279:string)
        n321 = call "Convert to Dynamic Data9"("Double"=w276) -> ("Dynamic Data Type"=w296:dynamicdata)  [unwired: 3 in]
        n322 = call "Convert to Dynamic Data10"("Double"=w277) -> ("Dynamic Data Type"=w297:dynamicdata)  [unwired: 3 in]
        n323 = call "Convert to Dynamic Data6"("Double"=w292) -> ("Dynamic Data Type"=w293:dynamicdata)  [unwired: 3 in]
        n324 = call "Convert to Dynamic Data7"("Double"=w275) -> ("Dynamic Data Type"=w294:dynamicdata)  [unwired: 3 in]
        n325 = call "Convert to Dynamic Data8"("Double"=w274) -> ("Dynamic Data Type"=w295:dynamicdata)  [unwired: 3 in]
        n326 = Concatenate Strings(w279, "\\data.lvm" ("string")) -> (w282:string)
        n327 = String To Path(string=w282) -> (path=w283:path)
        n328 = Merge Signals(w293, w294, w295, w296, w297) -> (w298:dynamicdata)
        n329 = xnode ("Set Dynamic Data Attributes")("Signals In"=w298) -> ("Signals Out"=w284:dynamicdata, "error out"=w286:errorcluster)  [unwired: 4 in]
        n330 = xnode ("Set Dynamic Data Attributes")("Signals In"=w284, "error in"=w286) -> ("Signals Out"=w285:dynamicdata, "error out"=w287:errorcluster)  [unwired: 3 in]
        n331 = xnode ("Set Dynamic Data Attributes")("Signals In"=w285, "error in"=w287) -> ("Signals Out"=w299:dynamicdata, "error out"=w288:errorcluster)  [unwired: 3 in]
        n332 = xnode ("Set Dynamic Data Attributes")("Signals In"=w299, "error in"=w288) -> ("Signals Out"=w300:dynamicdata, "error out"=w289:errorcluster)  [unwired: 3 in]
        n333 = xnode ("Set Dynamic Data Attributes")("Signals In"=w300, "error in"=w289) -> ("Signals Out"=w290:dynamicdata, "error out"=w291:errorcluster)  [unwired: 3 in]
        n334 = call "Write To Measurement File2"("Signals"=w290, "Enable"=w278, "error in (no error)"=w291, "Filename"=w283) -> ()  [unwired: 13 in, 3 out]
      }
    }
  }
  n335 = disable-structure shown="Disabled" {
    frame Disabled {
    }
    frame Enabled {
    }
  }
  "velocidade" <- "velocidade 2"
